vi "Join HDC Bank3 DIO.vi"(1 "IN 7:4":fxp<+,4,4> format="%04b", 2 "IN 3:0":fxp<+,4,4> format="%04b") -> (0 "OUT 7:0":u8 format="%08b")   [LabVIEW 2013]
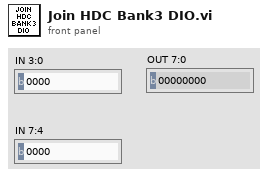
[diagram p1: front panel]
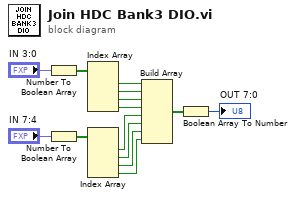
[diagram p0: block diagram]
diagram:
  n1 = Number To Boolean Array(number="IN 3:0") -> (Boolean array=w12:bool[])
  n2 = Number To Boolean Array(number="IN 7:4") -> (Boolean array=w11:bool[])
  n3 = Index Array(array=w12) -> (element #1=w10:bool, element #2=w9:bool, element #3=w8:bool, element #4=w7:bool)  [unwired: 4 in]
  n4 = Index Array(array=w11) -> (element #1=w4:bool, element #2=w3:bool, element #3=w2:bool, element #4=w1:bool)  [unwired: 4 in]
  n5 = Build Array(w10, w9, w8, w7, w4, w3, w2, w1) -> (w6:bool[])
  n6 = Boolean Array To Number(Boolean array=w6) -> (number=→"OUT 7:0":u8)
